vi "Create Subscriber.vi"(8 "error in (no error)":errorcluster, 9 "Default Value":dbl, 10 "Name":string, 11 "CIFTag in":refnum<class "CIFTagDouble.lvclass">) -> (0 "error out":errorcluster, 3 "CIFTag out":refnum<class "CIFTagDouble.lvclass">)   [LabVIEW 2021, in "CIFTagDouble.lvclass"]
uses:
  CIFTagDouble.lvclass
  D:/dev/CIF-LVCore/src/CIFUtilities/CIFChannels/CIFChannels.lvclass
  D:/dev/CIF-LVCore/src/Channels/CIFTag/CIFTag/CIFTag.lvclass
  CIFUtilities/CIFChannels/Typedef/Direction.ctl
  CIFUtilities/CIFChannels/Typedef/Disconnect Behavior.ctl
  CIFUtilities/CIFChannels/Typedef/Channel State.ctl
  CIFUtilities/CIFChannels/CIFChannels.lvclass/CIFChannels.ctl
  CIFTagDouble.lvclass/CIFTagDouble.ctl
  CIFTag/CIFTag.lvclass/CIFTag.ctl
  175b5bb0-395a-4b4a-8cf4-aadf4605253d.vi
  72532a7b-835d-4d7a-8c97-ceeadf54b86e.vi
  CIFUtilities/CIFChannels/Accessors/Write Channel State.vi
  CIFTag/Accessors/Write CIF Channel.vi
  CIFUtilities/CIFChannels/Accessors/Write Channel Class.vi
  CIFUtilities/CIFChannels/Accessors/Write Direction.vi
  CIFUtilities/CIFChannels/Accessors/Write Disconnect Behavior.vi
  CIFUtilities/CIFChannels/Accessors/Write Name.vi
  <vilib>/CIFChannels/SubVIs/Add Error.vi
  175b5bb0-395a-4b4a-8cf4-aadf4605253d.vi/c28b0ead-42ad-4072-80a2-aca7f2bd7ce3.vi
  <vilib>/CIFChannels/SubVIs/CIFServices Fill In Error Info Ex.vi
  <vilib>/CIFChannels/SubVIs/Get dll Path.vi
  72532a7b-835d-4d7a-8c97-ceeadf54b86e.vi/4bc1c15b-36ab-481f-b8dd-c64075ce723a.vi
  <vilib>/CIFChannels/SubVIs/Append Error Location.vi
  <vilib>/Utility/LVClass/Get LV Class Name.vi
  CIFUtilities/CIFChannels/CIFChannels.lvclass
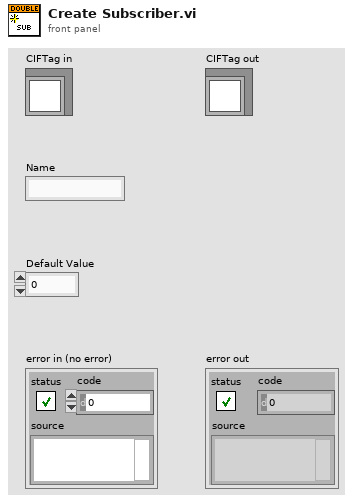
[diagram p1: front panel]
types:
  T1 = typedef "CIFChannels.lvclass/Channel State.ctl" = enum16{"Creating", "Disconnected", "Connecting", "Connected", "Destroying"}
  T2 = typedef "CIFChannels.lvclass/Disconnect Behavior.ctl" = enum16{"Default value", "Last value", "Error with default"}
  T3 = typedef "CIFChannels.lvclass/Direction.ctl" = enum16{"Publisher", "Subscriber"}
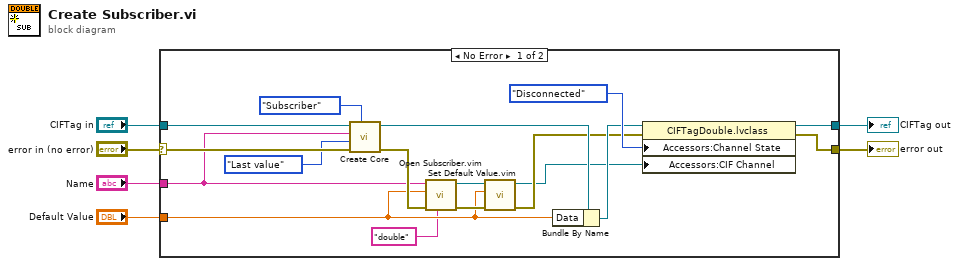
[diagram p0: block diagram]
diagram:
  n1 = case shown="No Error" "error in (no error)" {
    selector: "error in (no error)" -> [w21 w25]
    tunnel: [w18 w25] -> w4
    tunnel: [w14 w24] -> w5
    tunnel: "CIFTag in" -> [w23 w24]
    tunnel: "Name" -> [w7 _]
    tunnel: "Default Value" -> [w9 _]
    frame No Error {
      n2 = call "Create Core.vi"("Direction"=Direction."Subscriber", "error in (no error)"=w21, "Disconnect Behavior"=Disconnect_Behavior."Last value", "Name"=w7, "CIFChannels in"=w23) -> ("error out"=w17:errorcluster, "CIFChannels out"=w16:refnum<class "CIFTagDouble.lvclass">)  [unwired: 5 in]
      n3 = call "Open Subscriber.vim"("Channel Type Description"="double", "error in"=w17, "Input Type"=w9, "Channel Name"=w7) -> ("error out"=w13:errorcluster, "CIF Channel"=w12:refnum<k21>)  [unwired: 6 in]
      n4 = call "Set Default Value.vim"("error in"=w13, "Data in"=w9, "CIF Channel in"=w12) -> ("error out"=w11:errorcluster, "CIF Channel out"=w10:refnum<k21>)  [unwired: 7 in]
      n5 = Bundle By Name(cluster=w16, "Data"=w9) -> (w15:refnum<class "CIFTagDouble.lvclass">)
      n6 = property class="CIFTagDouble.lvclass"(reference=w15, error in=w11, "Accessors:Channel State"=Channel_State."Disconnected" ("Channel State"), "Accessors:CIF Channel"=w10) -> (reference out=w14:refnum<class "CIFTagDouble.lvclass">, error out=w18:errorcluster)
    }
    frame Error {
    }
  }
  "error out" <- w4
  "CIFTag out" <- w5
